vi "Global_SEN Write_Data.vi"() -> ()   [LabVIEW 2017]
uses:
  startup.rtexe/CLUSTER_Drive_Motion Profile Arrays.ctl
  startup.rtexe/CLUSTER_Drive_Point Specification.ctl
panel:
  in  "Dashboard_SEN_MotionProfiles":T1
  # "The Names of the Data items in the Global Variable MUST describe who the Single Writer is\nNaming Convention of all Data Items is:   Lib Name_Loop Name (SM or SEN or ACT)_Data Name\nExample   Drive_ACT_X axis;  GameController_SEN_JoystickLeft;  Hopper_SM_AgitatorSpeed"
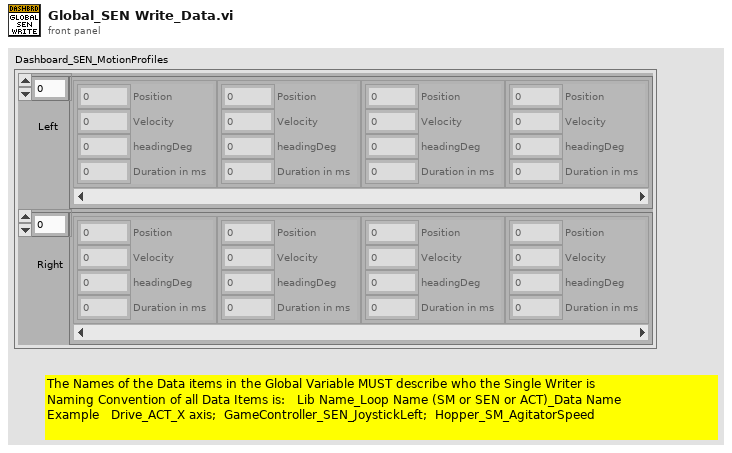
[diagram p1: front panel]
types:
  T1 = typedef "CLUSTER_Drive_Motion Profile Arrays.ctl" = cluster{"Left":T2[], "Right":T2[]}
  T2 = typedef "CLUSTER_Drive_Point Specification.ctl" = cluster{"Position":dbl, "Velocity":dbl, "headingDeg":dbl, "Duration in ms":i32}
diagram:
